vi "item selection selection force selection.vi"(8 "error in (no error)":errorcluster, 10 "Selection States":bool[](array[boolean]), 11 "Loop data":T1) -> (0 "error out":errorcluster, 3 "Loop data":T1)   [LabVIEW 2020, in "UI_ItemSelect.lvlib"]
uses:
  UI_ItemSelect.lvlib
  Tree item select loop data.ctl
  Item select ref type.ctl
  Tree item loop data.ctl
  Tree item selection indices.ctl
  checkbox state.ctl
  item select tree lock states.ctl
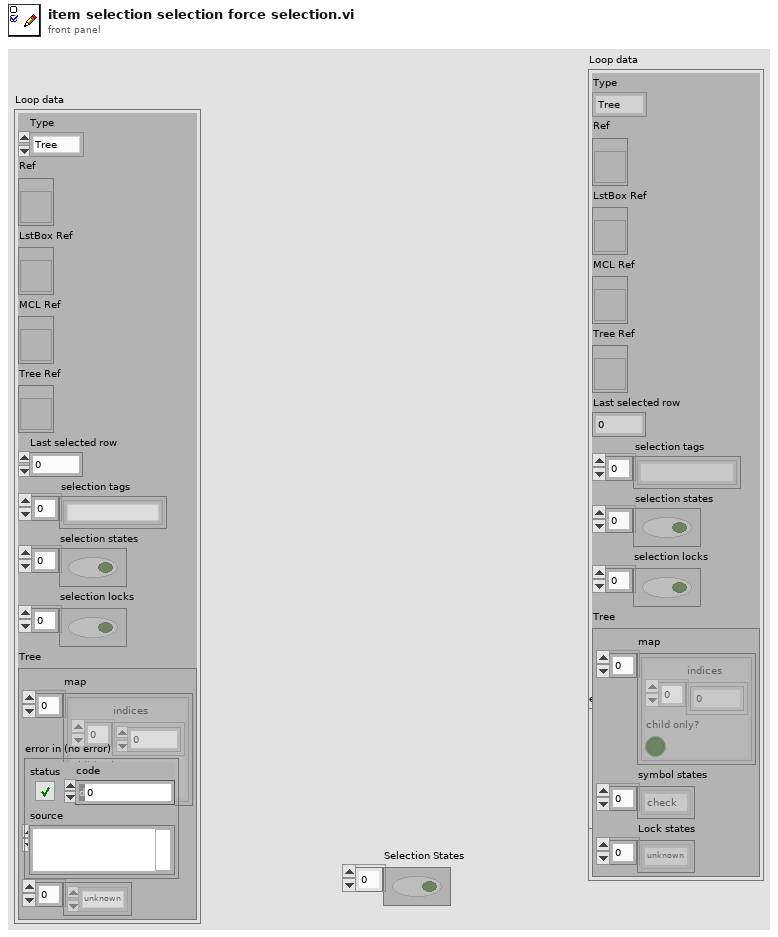
[diagram p1: front panel]
types:
  T1 = typedef "UI_ItemSelect.lvlib/Tree item select loop data.ctl" = cluster{"Type":T2, "Ref":refnum<vi>, "LstBox Ref":refnum<vi>, "MCL Ref":refnum<vi>, "Tree Ref":refnum<vi>, "Last selected row":i32, "selection tags":string[], "selection states":bool[], "selection locks":bool[], "Tree":T3}
  T2 = typedef "UI_ItemSelect.lvlib/Item select ref type.ctl" = enum16{"Tree", "MCL", "ListBox"}
  T3 = typedef "UI_ItemSelect.lvlib/Tree item loop data.ctl" = cluster{"map":T4[], "symbol states":T5[], "Lock states":T6[]}
  T4 = typedef "UI_ItemSelect.lvlib/Tree item selection indices.ctl" = cluster{"indices":i32[], "child only?":bool}
  T5 = typedef "UI_ItemSelect.lvlib/checkbox state.ctl" = enum16{"unknown", "check", "some", "no check"}
  T6 = typedef "UI_ItemSelect.lvlib/item select tree lock states.ctl" = enum16{"unknown", "locked", "unlocked"}
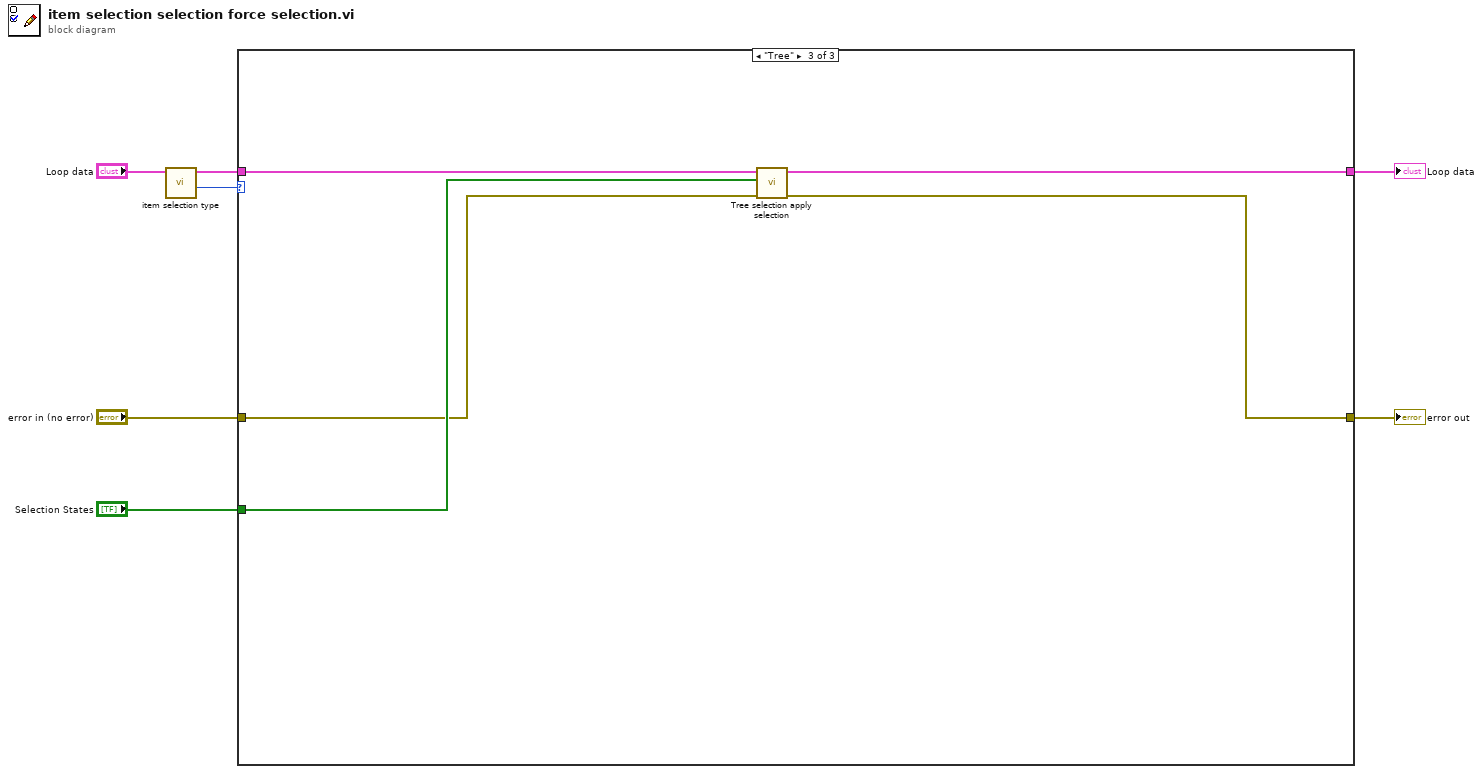
[diagram p0: block diagram]
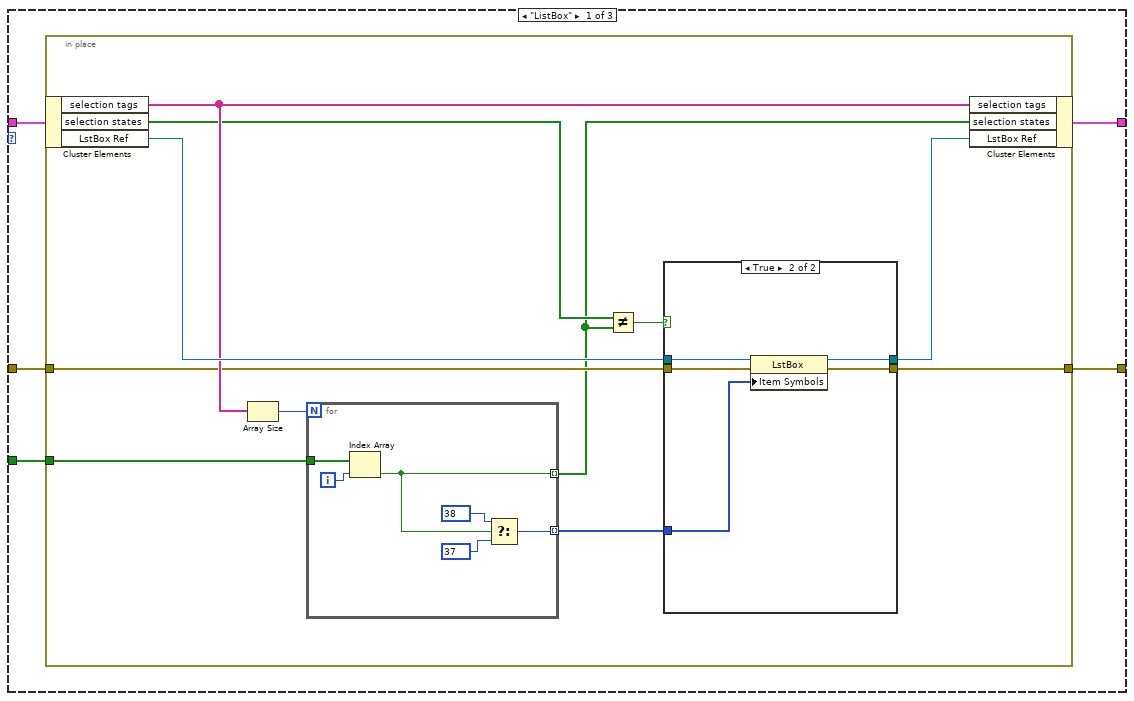
[diagram p2: hidden frame]
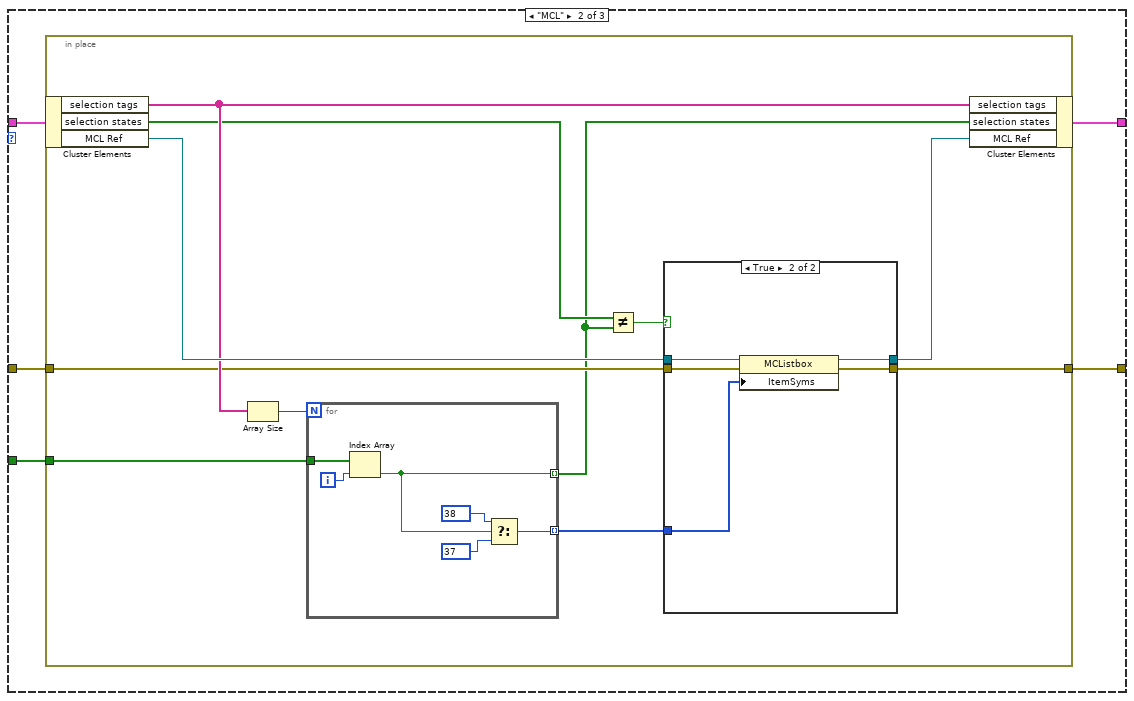
[diagram p4: hidden frame]
diagram:
  n1 = call "item selection type.vi"("Loop data"="Loop data") -> ("Type"=w4:T2, "Loop data"=w5:T1)  [unwired: 9 in]
  n2 = case shown="\"Tree\"" w4 {
    tunnel: "Selection States" -> [w12 w41 w68]
    tunnel: w5 -> [w11 w40 w70]
    tunnel: "error in (no error)" -> [w10 w39 w67]
    tunnel: [w9 w38 w66] -> w2
    tunnel: [w8 w37 w69] -> w1
    frame "ListBox" {
      n3 = in-place {
        in-place-border: w12 -> [w14]
        in-place-border: w10 -> [w17]
        in-place-border: [w15] -> w9
        n4 = in-place-cluster #1(w11) -> ("selection tags"=w22:string[], "selection states"=w19:bool[], "LstBox Ref"=w23:refnum<vi>)
        n5 = Array Size(array=w22) -> (size(s)=w21:i32)
        n6 = for {
          N: w21 -> [_]
          tunnel: w14 -> [w36]
          tunnel: [w32] -> w20 mode=indexing
          tunnel: [w31] -> w13 mode=indexing
          i -> [w35]
          n7 = Index Array(array=w36, index=w35) -> (element=w31:bool)
          n8 = Select(t=38, s=w31, f=37) -> (s? t:f=w32:i32)
        }
        n9 = Not Equal?(x=w19, y=w13) -> (x != y?=w18:bool)
        n10 = case shown="True" w18 {
          tunnel: w23 -> [w25 w30]
          tunnel: w20 -> [_ w29]
          tunnel: w17 -> [w24 w28]
          tunnel: [w25 w27] -> w16
          tunnel: [w24 w26] -> w15
          frame False {
          }
          frame True {
            n11 = property class="LstBox"(reference=w30, error in=w28, "Item Symbols"=w29) -> (reference out=w27:refnum<vi>, error out=w26:errorcluster)
          }
        }
        n12 = in-place-cluster #1("selection tags"=w22, "selection states"=w13, "LstBox Ref"=w16) -> (w8:T1)
      }
    }
    frame "MCL" {
      n13 = in-place {
        in-place-border: w41 -> [w43]
        in-place-border: w39 -> [w46]
        in-place-border: [w44] -> w38
        n14 = in-place-cluster #2(w40) -> ("selection tags"=w51:string[], "selection states"=w48:bool[], "MCL Ref"=w52:refnum<vi>)
        n15 = Array Size(array=w51) -> (size(s)=w50:i32)
        n16 = for {
          N: w50 -> [_]
          tunnel: w43 -> [w65]
          tunnel: [w61] -> w49 mode=indexing
          tunnel: [w60] -> w42 mode=indexing
          i -> [w64]
          n17 = Index Array(array=w65, index=w64) -> (element=w60:bool)
          n18 = Select(t=38, s=w60, f=37) -> (s? t:f=w61:i32)
        }
        n19 = Not Equal?(x=w48, y=w42) -> (x != y?=w47:bool)
        n20 = case shown="True" w47 {
          tunnel: w52 -> [w54 w59]
          tunnel: w49 -> [_ w58]
          tunnel: w46 -> [w53 w57]
          tunnel: [w54 w56] -> w45
          tunnel: [w53 w55] -> w44
          frame False {
          }
          frame True {
            n21 = property class="MCListbox"(reference=w59, error in=w57, "ItemSyms"=w58) -> (reference out=w56:refnum<vi>, error out=w55:errorcluster)
          }
        }
        n22 = in-place-cluster #2("selection tags"=w51, "selection states"=w42, "MCL Ref"=w45) -> (w37:T1)
      }
    }
    frame "Tree" {
      n23 = call "Tree selection apply selection.vi"("error in (no error)"=w67, "Selection States"=w68, "Loop data"=w70) -> ("error out"=w66:errorcluster, "Loop data"=w69:T1)  [unwired: 7 in]
    }
  }
  "error out" <- w2
  "Loop data" <- w1
